vi "Chol33.vi"(11 "Matrix In":fxp<+,64,57>[](array[numeric])=[0.0, 0.0, 0.0, 0.0, 0.0, 0.0, 0.0, 0.0, 0.0]) -> (3 "L":fxp<+,64,57>[](array[numeric]) format="%.25g")   [LabVIEW 2014]
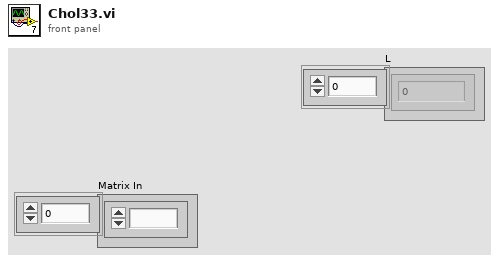
[diagram p1: front panel]
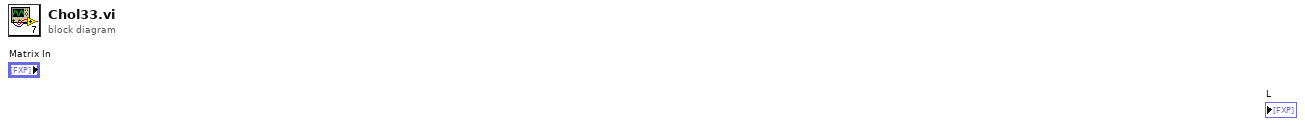
[diagram p0: block diagram]
diagram:
